vi "Read Primary Conditions.vi"(10 "amps?":bool caption="Amps", 11 "magarray":T1(array[cluster])) -> (0 "levels":cluster{"LHelevel":dbl, "LNlevel":dbl}, 1 "temp":dbl caption="Temperature", 2 "rate":dbl caption="Rate", 3 "currentfield":dbl caption="Current Field", 4 "persistent?":bool caption="Persistent")   [LabVIEW 2009, in "Magnet.lvclass"]
uses:
  Magnet.lvclass
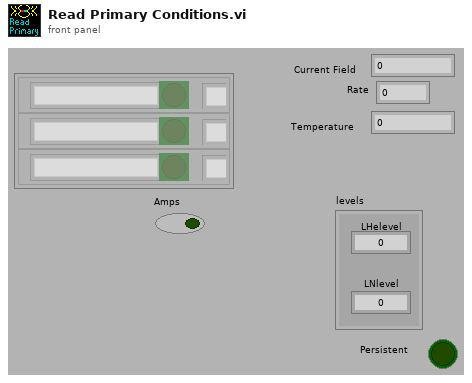
[diagram p1: front panel]
types:
  T1 = cluster{"name":string, "on?":bool, "abbrev":string}[]
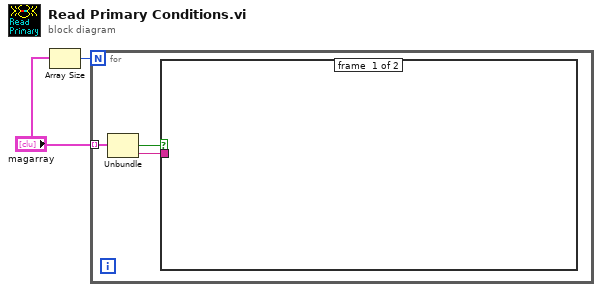
[diagram p0: block diagram]
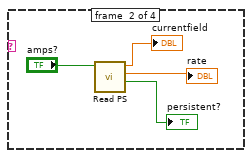
[diagram p3: hidden frame]
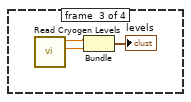
[diagram p4: hidden frame]
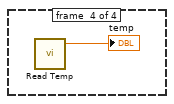
[diagram p5: hidden frame]
diagram:
  n1 = Array Size(array="magarray") -> (size(s)=w2:i32)
  n2 = for {
    N: w2 -> [_]
    tunnel: "magarray" -> [w5] mode=indexing
    n3 = Unbundle(w5) -> ("on?"=w3:bool, "abbrev"=w4:string)  [unwired: 1 out]
    n4 = case shown="True" w3 {
      tunnel: w4 -> [_ w6]
      frame #0 {
      }
      frame #1 {
        n5 = case shown="\"TC\"" w6 {
          frame #0 {
          }
          frame #1 {
            n6 = call "Read PS.vi"("amps?"="amps?") -> ("persistent?"=→"persistent?":bool, "rate"=→"rate":dbl, "currentfield"=→"currentfield":dbl)  [unwired: 8 out]
          }
          frame #2 {
            n7 = call "Read Cryogen Levels.vi"() -> ("LNlevel"=w12:dbl, "LHelevel"=w13:dbl)  [unwired: 10 out]
            n8 = Bundle("LHelevel"=w13, "LNlevel"=w12) -> (→"levels":cluster{"LHelevel":dbl, "LNlevel":dbl})  [unwired: 1 out]
          }
          frame #3 {
            n9 = call "Read Temp.vi"() -> ("temp"=→"temp":dbl)  [unwired: 7 out]
          }
        }
      }
    }
  }
